vi "format_time.vi"(1 "extra":string=".txt", 2 "format":string="%Y%m%d %H%M%S") -> (0 "output":string)   [LabVIEW 2017]
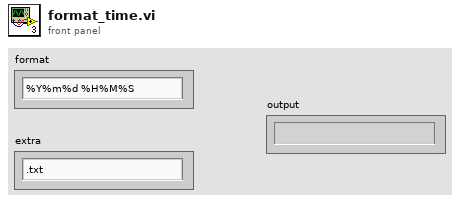
[diagram p1: front panel]
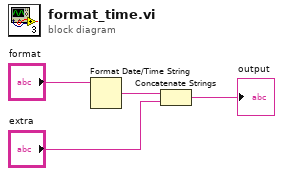
[diagram p0: block diagram]
diagram:
  n1 = Format Date/Time String(time format string (%c)="format") -> (date/time string=w3:string)  [unwired: 2 in]
  n2 = Concatenate Strings(w3, "extra") -> (→"output":string)
